vi "SR_MU-Add_Op.vi"(8 "Init":bool, 9 "Latitude In":dbl, 10 "Longitude In":dbl, 11 "Mission In":T1[](array[typedef]) {"GPS Longitude" format="%.6g"; "GPS Latitude" format="%.6g"}) -> (1 "Add?":bool, 2 "Output":T1 {"GPS Longitude" format="%.6g"; "GPS Latitude" format="%.6g"}, 3 "Mission Out":T1[](array[typedef]) {"GPS Longitude" format="%.6g"; "GPS Latitude" format="%.6g"})   [LabVIEW 2015, in "Shore Library.lvlib"]
uses:
  Shore Library.lvlib
  RDS Mission Controller Actor/MissionOp.ctl
  RDS Mission Controller Actor/RDS Mission Controller Actor.lvlib
panel:
  in  "btn_cancel":bool
  in  "btn_add":bool
  in  "Longitude":dbl
  in  "Latitude":dbl
  in  "Throttle":i16
  in  "Duration (s)":u16
  in  "MissionOp Type":T2(ring)
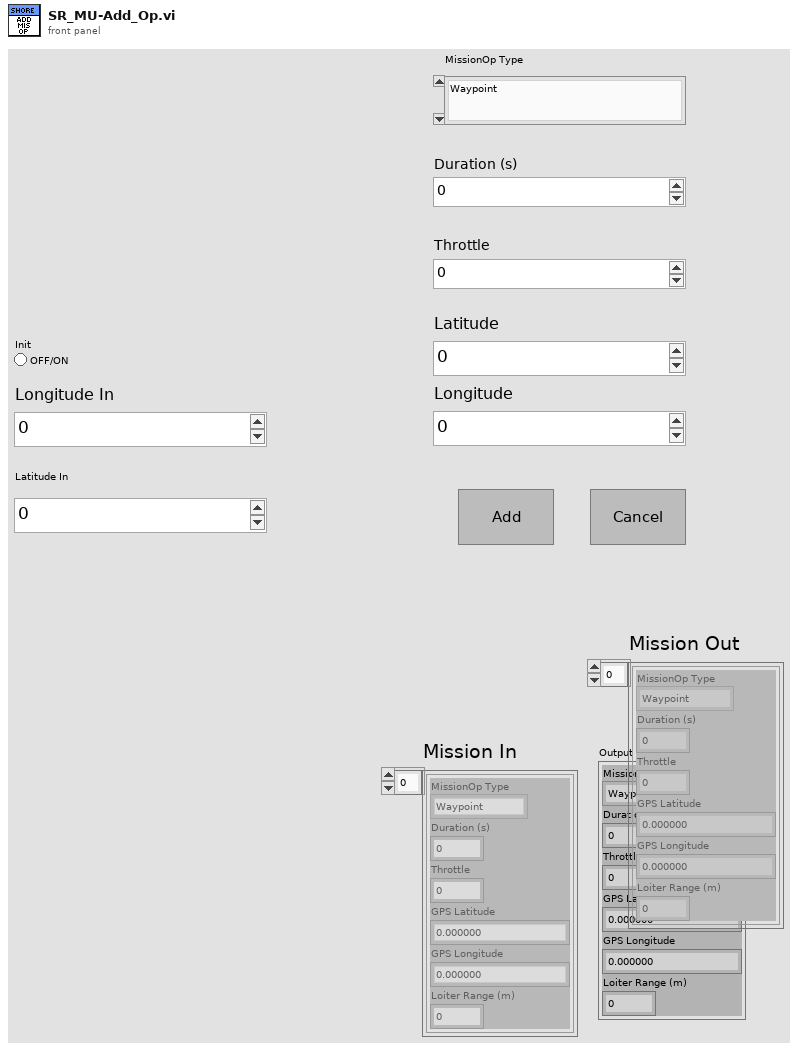
[diagram p1: front panel]
types:
  T1 = typedef "RDS Mission Controller Actor.lvlib/MissionOp.ctl" = cluster{"MissionOp Type":enum16{"Waypoint", "Loiter", "Wait", "Deploy AIP", "Stow AIP"}, "Duration (s)":u16, "Throttle":i16, "GPS Latitude":dbl, "GPS Longitude":dbl, "Loiter Range (m)":u16}
  T2 = enum16{"Waypoint", "Loiter", "Wait", "Deploy AIP", "Stow AIP"}
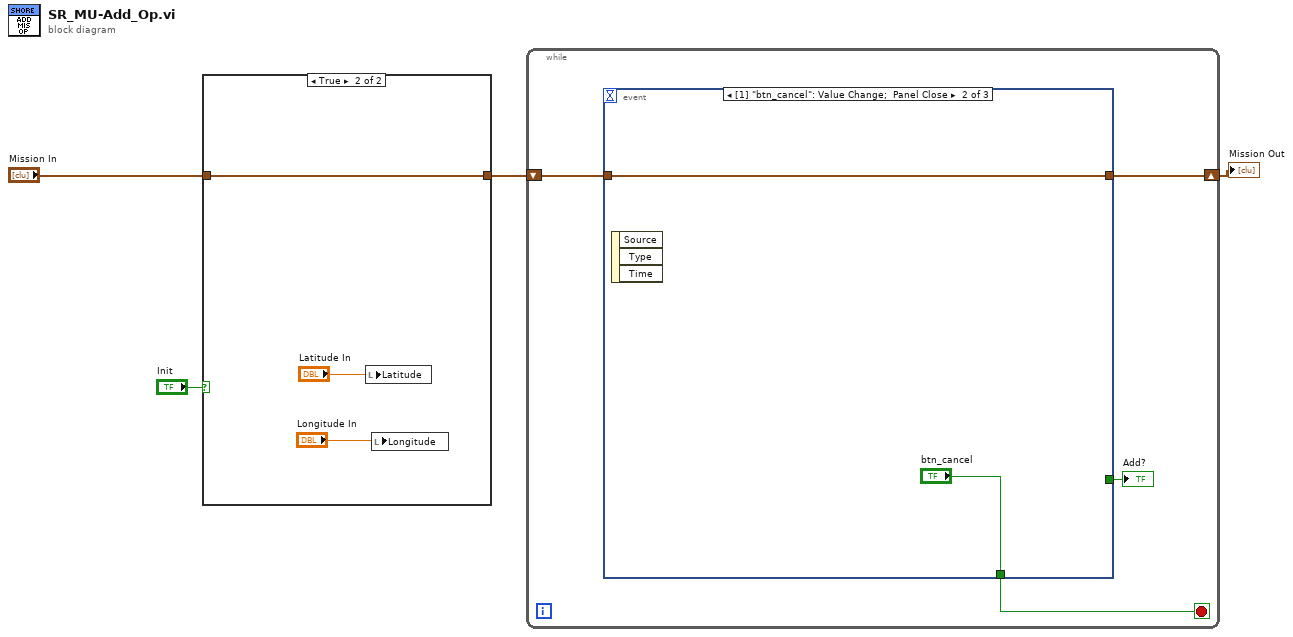
[diagram p0: block diagram]
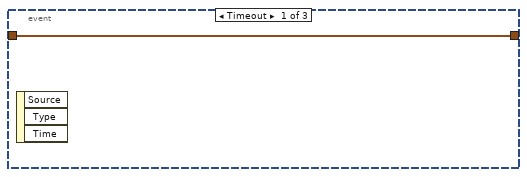
[diagram p3: hidden frame]
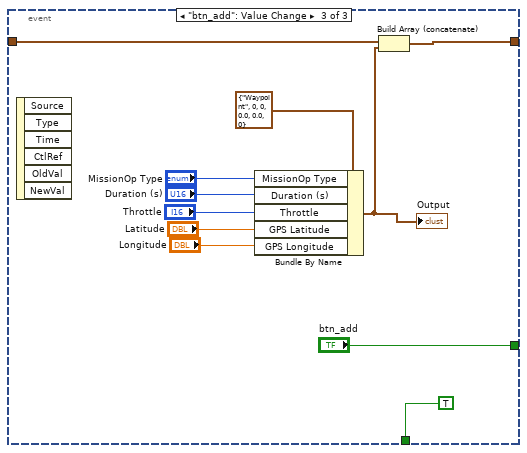
[diagram p4: hidden frame]
diagram:
  n1 = case shown="True" "Init" {
    tunnel: [w5 w6] -> w2
    tunnel: "Mission In" -> [w5 w6]
    frame False {
    }
    frame True {
      n2 = local write "Latitude"("Latitude In") -> ()
      n3 = local write "Longitude"("Longitude In") -> ()
    }
  }
  n4 = while {
    shift-right: [w9] -> w4
    shift-left: w2 -> [w10]
    stop <- w12 stop-if-true
    n5 = event shown="[1] \"btn_cancel\": Value Change;  Panel Close" {
      selector: _ -> [_ _ _]
      dyn-events: _ -> [_ _ _]
      timeout: _ -> [_ _ _]
      tunnel: [_ _ "btn_add"] -> w11
      tunnel: [_ "btn_cancel" TRUE ("btn_add")] -> w12
      tunnel: w10 -> [w13 w14 w18]
      tunnel: [w13 w14 w16] -> w9
      event Timeout {
        n6 = event-data() -> ()  [unwired: 1 in, 3 out]
      }
      event "btn_cancel": Value Change; Panel Close {
        n7 = event-data() -> ()  [unwired: 1 in, 3 out]
      }
      event "btn_add": Value Change {
        n8 = event-data() -> ()  [unwired: 1 in, 6 out]
        n9 = Bundle By Name(cluster=T1 {"MissionOp Type"=enum."Waypoint", "Duration (s)"=0, "Throttle"=0, "GPS Latitude"=0.0, "GPS Longitude"=0.0, "Loiter Range (m)"=0} ("MissionOp"), "MissionOp Type"="MissionOp Type", "Duration (s)"="Duration (s)", "Throttle"="Throttle", "GPS Latitude"="Latitude", "GPS Longitude"="Longitude") -> (w17:T1)
        "Output" <- w17
        n10 = Build Array (concatenate)(w18, w17) -> (w16:T1[])
      }
    }
    "Add?" <- w11
  }
  "Mission Out" <- w4
